vi "_builtins_visible_index.vi"(8 "error in (no error)":errorcluster, 10 "index display":enum8{"hide", "show"}(ring), 11 "GObject in":refnum<vi>) -> (0 "error out":errorcluster, 1 "was index visible?":enum8{"hide", "show"}(ring), 2 "has index display?":bool, 3 "GObject out":refnum<vi>)   [LabVIEW 2019, in "Script.lvlib"]
doc: "Shows or hides the index display on array controls or constants.\n\nCreated by: Ryan Pacini"
uses:
  Script.lvlib
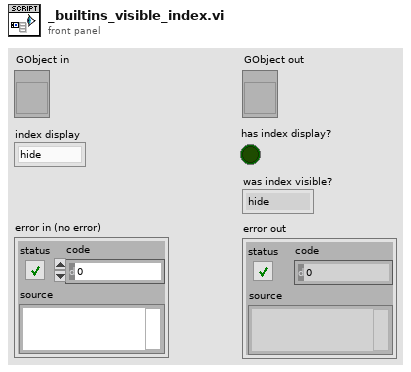
[diagram p1: front panel]
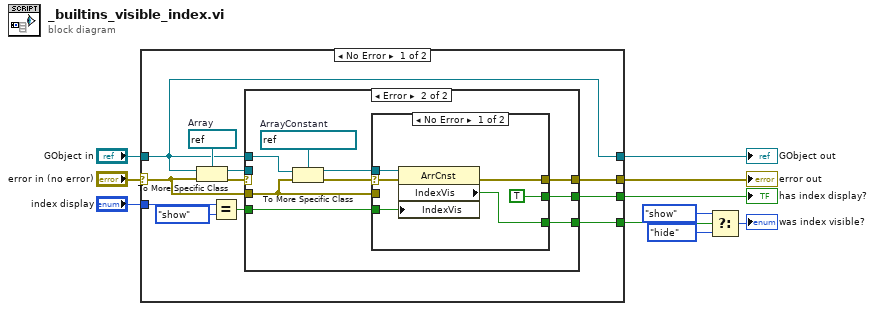
[diagram p0: block diagram]
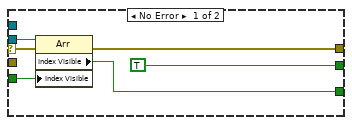
[diagram p2: hidden frame]
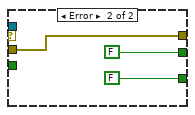
[diagram p3: hidden frame]
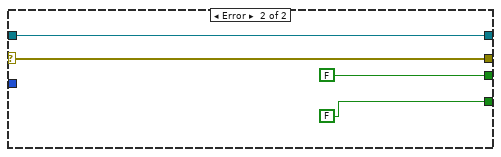
[diagram p4: hidden frame]
diagram:
  n1 = case shown="No Error" "error in (no error)" {
    selector: "error in (no error)" -> [w21 w48]
    tunnel: "index display" -> [w13 _]
    tunnel: [w15 FALSE ("Visible")] -> w5
    tunnel: [w16 w48] -> w4
    tunnel: "GObject in" -> [w14 w49]
    tunnel: [w14 w49] -> w2
    tunnel: [w17 FALSE] -> w1
    frame No Error {
      w18 = refnum<vi> refnum  # Array
      n2 = To More Specific Class(target class=w18, reference=w14, error in=w21) -> (specific class reference=w19:refnum<vi>, error out=w20:errorcluster)
      n3 = Equal?(x=w13, y=enum8{"hide", "show"}."show") -> (x = y?=w12:bool)
      n4 = case shown="Error" w20 {
        selector: w20 -> [w27 _]
        tunnel: w19 -> [w26 _]
        tunnel: w21 -> [_ w28]
        tunnel: [w25 w32] -> w16
        tunnel: [TRUE w36] -> w17
        tunnel: [w23 w30] -> w15
        tunnel: w12 -> [w22 w29]
        tunnel: w14 -> [_ w34]
        frame No Error {
          n5 = property class="Arr"(reference=w26, error in=w27, "Index Visible"=w22) -> (error out=w25:errorcluster, "Index Visible"=w23:bool)  [unwired: 1 out]
        }
        frame Error {
          w33 = refnum<vi> refnum  # ArrayConstant
          n6 = To More Specific Class(target class=w33, reference=w34, error in=w28) -> (specific class reference=w31:refnum<vi>, error out=w35:errorcluster)
          n7 = case shown="No Error" w35 {
            selector: w35 -> [w41 _]
            tunnel: [TRUE FALSE] -> w36
            tunnel: [w40 w45] -> w32
            tunnel: w31 -> [w39 _]
            tunnel: [w38 FALSE ("IndexVis")] -> w30
            tunnel: w29 -> [w37 _]
            tunnel: w28 -> [_ w45]
            frame No Error {
              n8 = property class="ArrCnst"(reference=w39, error in=w41, "IndexVis"=w37) -> (error out=w40:errorcluster, "IndexVis"=w38:bool)  [unwired: 1 out]
            }
            frame Error {
            }
          }
        }
      }
    }
    frame Error {
    }
  }
  "error out" <- w4
  "GObject out" <- w2
  "has index display?" <- w1
  n9 = Select(t=enum8{"hide", "show"}."show" ("was inc/dec visible?"), s=w5, f=enum8{"hide", "show"}."hide" ("was inc/dec visible?")) -> (s? t:f=→"was index visible?":enum8{"hide", "show"})
